vi "Initialize.vi"(8 "error in (no error)":errorcluster, 9 "Send \"Connect client\"":bool=TRUE, 10 "Reset":bool=TRUE, 11 "RP Transceiver in":refnum<class "RP Transceiver.lvclass">) -> (0 "error out":errorcluster, 3 "RP Transceiver out":refnum<class "RP Transceiver.lvclass">)   [LabVIEW 2018, in "RP Transceiver.lvclass"]
uses:
  RP Transceiver.lvclass
  C:/github/NHMFL_Core/Libraries/Red Pitaya/RP Core/RP Instrument/RP Instrument.lvclass
  RP Transceiver.lvclass/RP Transceiver.ctl
  RP Instrument/RP Instrument.lvclass/RP Instrument.ctl
  Write Total decimation.vi
  RP Instrument/Write Decimation.vi
  RP Instrument/Write bytes per RX sample.vi
  RP Instrument/RP Instrument.lvclass
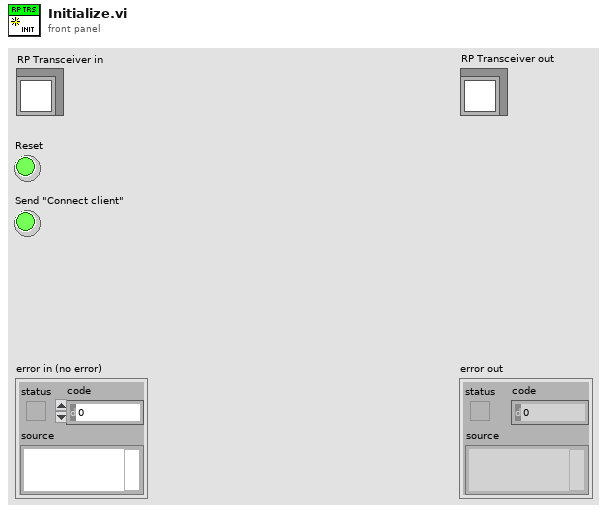
[diagram p1: front panel]
types:
  T1 = typedef "Receiver format.ctl" = enum16{"X-Y-F", "F-X-Y", "X-Y", "X"}
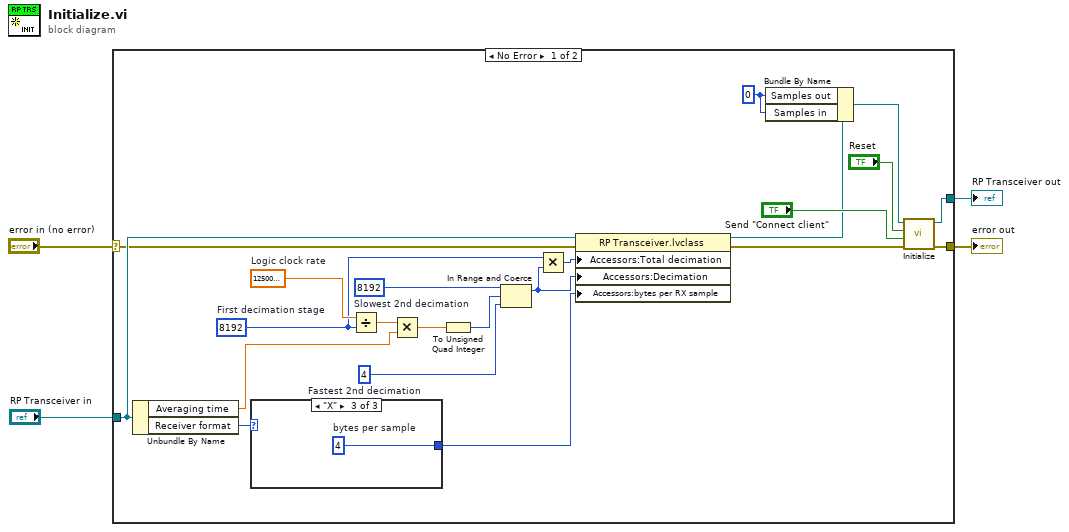
[diagram p0: block diagram]
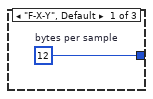
[diagram p2: hidden frame]
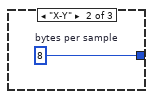
[diagram p3: hidden frame]
diagram:
  n1 = case shown="No Error" "error in (no error)" {
    selector: "error in (no error)" -> [w11 w31]
    tunnel: [w12 w31] -> w3
    tunnel: [w10 w30] -> w1
    tunnel: "RP Transceiver in" -> [w18 w30]
    frame No Error {
      w5 = u64 0 ("Samples in")
      w20 = u64 8192  # Slowest 2nd decimation
      w19 = u64 8192  # First decimation stage
      w23 = u64 4  # Fastest 2nd decimation
      w26 = 125000000.0  # Logic clock rate
      n2 = Unbundle By Name(w18) -> ("Averaging time"=w22:dbl, "Receiver format"=w8:T1)
      n3 = case shown="\"X\"" w8 {
        tunnel: [w27 w28 w29] -> w7
        frame "F-X-Y", Default {
          w27 = 12  # bytes per sample
        }
        frame "X-Y" {
          w28 = 8  # bytes per sample
        }
        frame "X" {
          w29 = 4  # bytes per sample
        }
      }
      n4 = Divide(x=w26, y=w19) -> (x/y=w21:dbl)
      n5 = Multiply(x=w21, y=w22) -> (x*y=w25:dbl)
      n6 = To Unsigned Quad Integer(1:w25) -> (0:w24:u64)
      n7 = In Range and Coerce(upper limit=w20, x=w24, lower limit=w23) -> (coerced(x)=w9:u64)  [unwired: 1 out]
      n8 = Multiply(x=w19, y=w9) -> (x*y=w17:u64)
      n9 = property class="RP Transceiver.lvclass"(reference=w18, error in=w11, "Accessors:Total decimation"=w17, "Accessors:Decimation"=w9, "Accessors:bytes per RX sample"=w7) -> (reference out=w14:refnum<class "RP Transceiver.lvclass">, error out=w13:errorcluster)
      n10 = Bundle By Name(cluster=w14, "Samples out"=w5, "Samples in"=w5) -> (w6:refnum<class "RP Transceiver.lvclass">)
      n11 = call-parent "Initialize.vi"("error in (no error)"=w13, "Send \"Connect client\""="Send \"Connect client\"", "Reset"="Reset", "RP Instrument in"=w6) -> ("error out"=w12:errorcluster, "RP Instrument out"=w10:refnum<class "RP Transceiver.lvclass">)  [unwired: 6 in]
    }
    frame Error {
    }
  }
  "error out" <- w3
  "RP Transceiver out" <- w1
